vi "To Black & White(SubVI).vi"(8 "error in (no error)":errorcluster, 10 "Range":cluster{"Lower value":sgl, "Upper value":sgl}={"Lower value"=180.0, "Upper value"=255.0}, 11 "Refnum in":T1) -> (0 "error out":errorcluster, 3 "Refnum out":T1)   [LabVIEW 2014]
uses:
  <vilib>/vision/Image Controls.llb/IMAQ Image.ctl
  <vilib>/vision/NI_Vision_Development_Module.lvlib
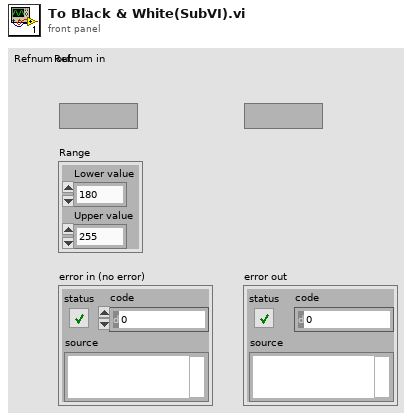
[diagram p1: front panel]
types:
  T1 = typedef "IMAQ Image.ctl" = refnum<image>
  T2 = typedef "Image Type" = u32
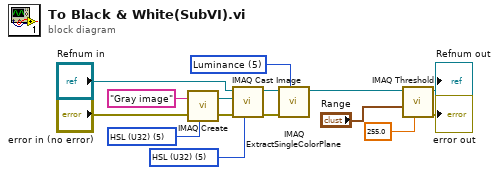
[diagram p0: block diagram]
diagram:
  w6 = T2 5 items=["Grayscale (U8)", "Grayscale (I16)", "Grayscale (SGL)", "Complex (CSG)", "RGB (U32)", "HSL (U32)", "RGB (U64)", "Grayscale (U16)"] ("Image Type")
  w4 = T2 5 items=["Grayscale (U8)", "Grayscale (I16)", "Grayscale (SGL)", "Complex (CSG)", "RGB (U32)", "HSL (U32)", "RGB (U64)", "Grayscale (U16)"] ("Image Type")
  w3 = 5 items=["Red", "Green", "Blue", "Hue", "Saturation", "Luminance", "Value", "Intensity"] ("Color Plane")
  n1 = call "IMAQ Create"("Image Name"="Gray image", "Image Type"=w4, "error in (no error)"="error in (no error)") -> ("New Image"=w1:T1, "error out"=w7:errorcluster)  [unwired: 2 in]
  n2 = call "IMAQ Cast Image"("Image Type"=w6, "error in (no error)"=w7, "Image Dst"=w1, "Image Src"="Refnum in") -> ("error out"=w8:errorcluster, "Image Dst Out"=w2:T1)  [unwired: 6 in]
  n3 = call "IMAQ ExtractSingleColorPlane"("Color Plane"=w3, "error in (no error)"=w8, "Image Src"=w2) -> ("Image Dst Out"=w13:T1)  [unwired: 7 in, 1 out]
  n4 = call "IMAQ Threshold"("Replace Value"=sgl 255.0, "Range"="Range", "Image Src"=w13) -> ("error out"=→"error out":errorcluster, "Image Dst Out"=→"Refnum out":T1)  [unwired: 7 in]
